vi "Cyl_Num.vi"(1 "CurrentCAD":fxp<+,18,11>) -> (0 "Cylinder_Num":u8)   [LabVIEW 2023]
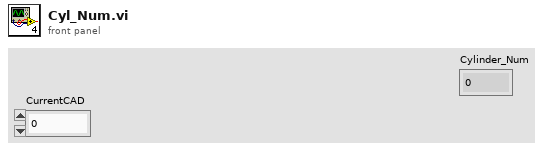
[diagram p1: front panel]
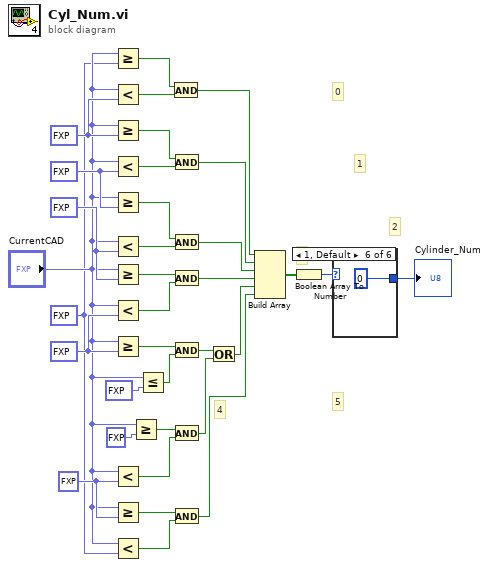
[diagram p0: block diagram]
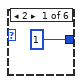
[diagram p2: hidden frame]
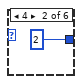
[diagram p3: hidden frame]
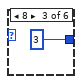
[diagram p4: hidden frame]
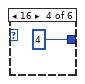
[diagram p5: hidden frame]
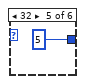
[diagram p6: hidden frame]
diagram:
  w13 = fxp<+,18,11> 30.0 ("y")
  w22 = fxp<+,18,11> 630.0 ("y")
  w25 = fxp<+,18,11> 510.0 ("y")
  w28 = fxp<+,18,11> 390.0 ("y")
  w29 = fxp<+,18,11> 270.0 ("y")
  w11 = fxp<+,18,11> 150.0 ("y")
  # "5"
  # "4"
  # "3"
  # "2"
  # "1"
  # "0"
  n1 = Greater Or Equal?(x="CurrentCAD", y=w11) -> (x >= y?=w34:bool)
  n2 = Less?(x="CurrentCAD", y=w29) -> (x < y?=w33:bool)
  n3 = Greater Or Equal?(x="CurrentCAD", y=w29) -> (x >= y?=w31:bool)
  n4 = Less?(x="CurrentCAD", y=w28) -> (x < y?=w30:bool)
  n5 = Greater Or Equal?(x="CurrentCAD", y=w28) -> (x >= y?=w27:bool)
  n6 = Less?(x="CurrentCAD", y=w25) -> (x < y?=w26:bool)
  n7 = Greater Or Equal?(x="CurrentCAD", y=w25) -> (x >= y?=w24:bool)
  n8 = Less?(x="CurrentCAD", y=w22) -> (x < y?=w23:bool)
  n9 = Greater Or Equal?(x="CurrentCAD", y=w22) -> (x >= y?=w20:bool)
  n10 = Less?(x="CurrentCAD", y=w13) -> (x < y?=w16:bool)
  n11 = Greater Or Equal?(x="CurrentCAD", y=w13) -> (x >= y?=w10:bool)
  n12 = Less?(x="CurrentCAD", y=w11) -> (x < y?=w9:bool)
  n13 = Greater Or Equal?(x="CurrentCAD", y=fxp<+,18,11> 0.0) -> (x >= y?=w17:bool)
  n14 = Less Or Equal?(x="CurrentCAD", y=fxp<+,18,11> 720.0) -> (x <= y?=w19:bool)
  n15 = And(x=w34, y=w33) -> (x .and. y?=w32:bool)
  n16 = And(x=w31, y=w30) -> (x .and. y?=w8:bool)
  n17 = And(x=w27, y=w26) -> (x .and. y?=w7:bool)
  n18 = And(x=w24, y=w23) -> (x .and. y?=w6:bool)
  n19 = And(x=w20, y=w19) -> (x .and. y?=w15:bool)
  n20 = And(x=w17, y=w16) -> (x .and. y?=w14:bool)
  n21 = And(x=w10, y=w9) -> (x .and. y?=w4:bool)
  n22 = Or(x=w15, y=w14) -> (x .or. y?=w5:bool)
  n23 = Build Array(w32, w8, w7, w6, w5, w4) -> (w3:bool[])
  n24 = Boolean Array To Number(Boolean array=w3) -> (number=w2:u8)
  n25 = case shown="1, Default" w2 {
    tunnel: [u8 1 u8 2 u8 3 u8 4 u8 5 u8 0] -> w1
    frame 2 {
    }
    frame 4 {
    }
    frame 8 {
    }
    frame 16 {
    }
    frame 32 {
    }
    frame 1, Default {
    }
  }
  "Cylinder_Num" <- w1
